vi "Configuration Files.vi"(8 "error in (no error)":errorcluster, 11 "Node Ptr":T3 format="%.0x") -> (0 "error out":errorcluster)   [LabVIEW 2020, in "Ballard ARINC 429 System Explorer.lvlib" / "Implementation.lvlib"]
uses:
  Implementation.lvlib
  <vilib>/NI VeriStand/Custom Device API/Custom Device Item Ref.ctl
  Types/Path Control.ctl
  Types/Browse Button.ctl
  Types/Configuration Files Page Data.ctl
  <vilib>/NI VeriStand/Custom Device API/Custom Device API.lvlib
  <vilib>/NI VeriStand/Custom Device Tools/Custom Device Utility Library/Custom Device Utility Library.lvlib
  Scripting/Ballard/Ballard ARINC 429 Scripting.lvlib
panel:
  in  "Refresh":bool
  in  "Parameters":T1
  in  "Hardware":T1
  in  "SHDocVw.IWebBrowser":refnum<k7>(container)
  in  "General Header":cluster{"Section Name":string}={"Section Name"="Ballard ARINC 429 - Configuration Files"}
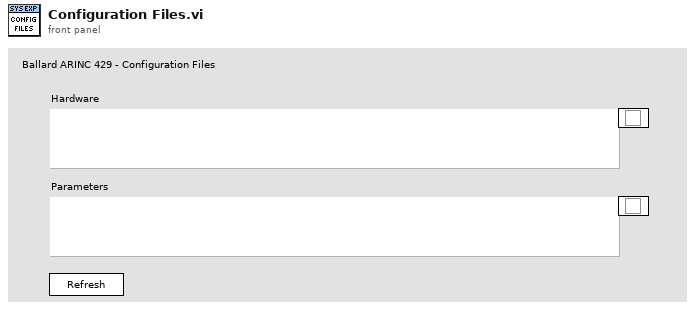
[diagram p1: front panel]
types:
  T1 = typedef "Ballard ARINC 429 System Explorer.lvlib/Implementation.lvlib/Path Control.ctl" = cluster{"file path":path, "Browse":T2}
  T2 = typedef "Ballard ARINC 429 System Explorer.lvlib/Implementation.lvlib/Browse Button.ctl" = bool
  T3 = typedef "Custom Device API.lvlib/Custom Device Item Ref.ctl" = u64
  T4 = typedef "Ballard ARINC 429 System Explorer.lvlib/Implementation.lvlib/Configuration Files Page Data.ctl" = cluster{"Hardware":T1, "Parameters":T1, "most recent parameters path":path, "most recent hardware path":path, "custom device ref":T3, "MD5 error":bool}
  T5 = typedef "Custom Device API.lvlib/Custom Device Commands.ctl" = enum16{"Default", "Item renamed", "Shutdown", "Dynamic button pressed"}
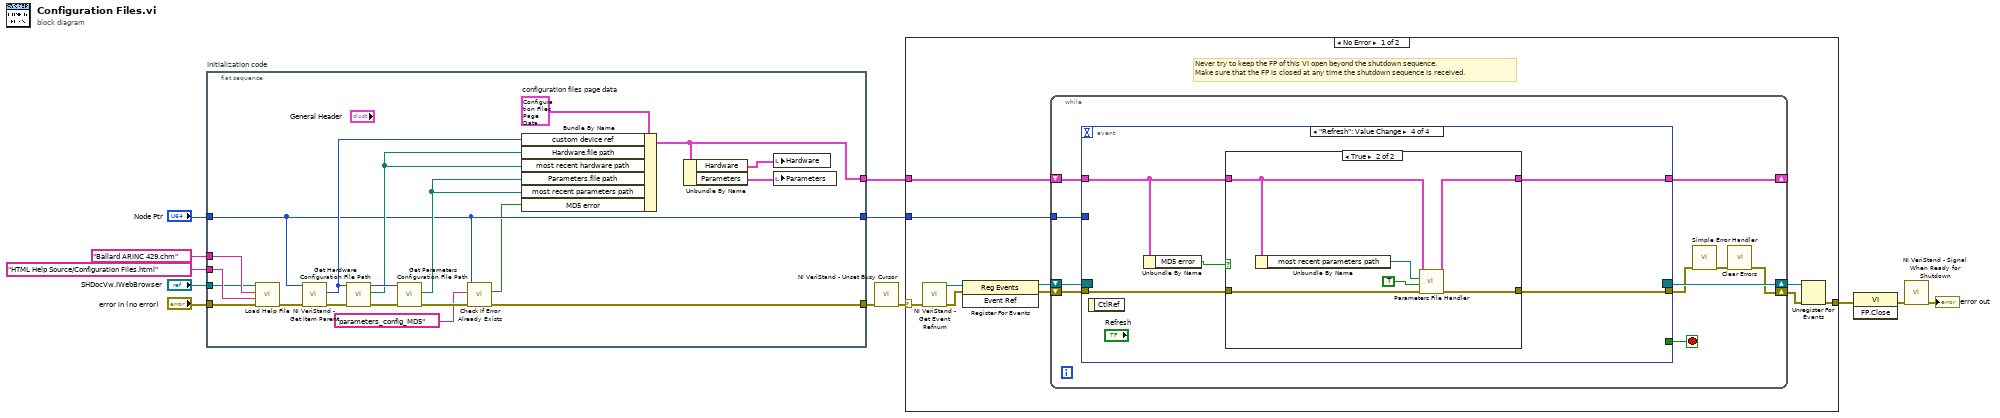
[diagram p0: block diagram]
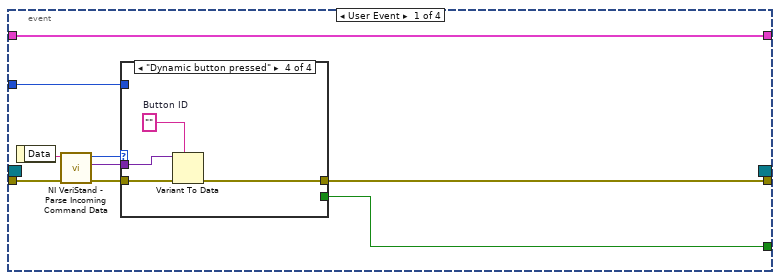
[diagram p2: hidden frame]
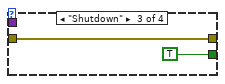
[diagram p5: hidden frame]
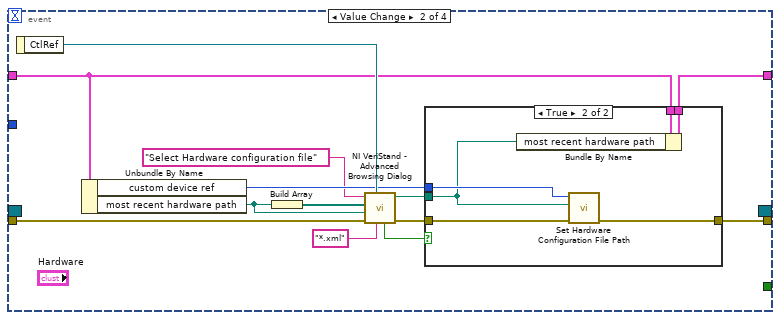
[diagram p6: hidden frame]
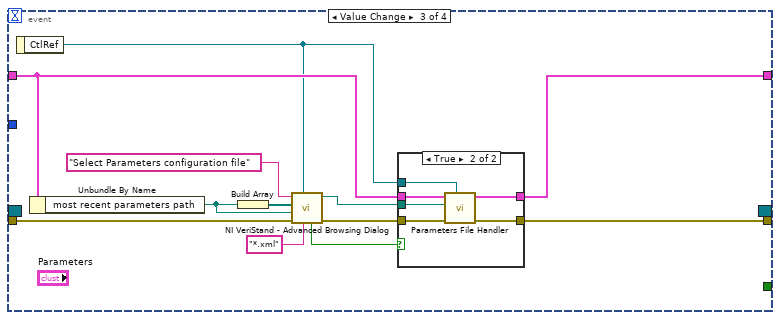
[diagram p8: hidden frame]
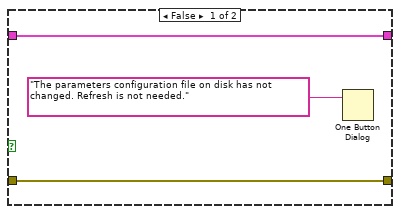
[diagram p10: hidden frame]
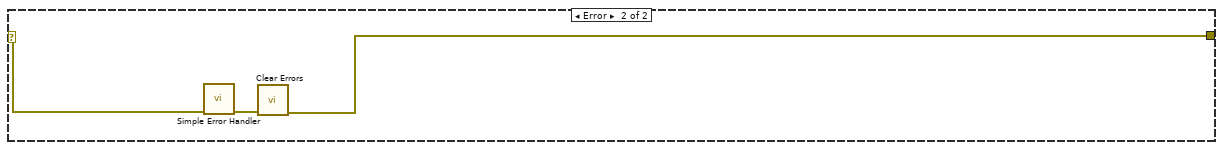
[diagram p11: hidden frame]
diagram:
  n1 = flat-sequence "Initialization code" {
    tunnel: "error in (no error)" -> [w32]
    tunnel: "Node Ptr" -> [w15]
    tunnel: [w16] -> w8
    tunnel: [w15] -> w5
    tunnel: "SHDocVw.IWebBrowser" -> [w20]
    tunnel: "HTML Help Source/Configuration Files.html" ("CD_CHM_Section") -> [w31]
    tunnel: "Ballard ARINC 429.chm" ("CD_CHM_FileName") -> [w30]
    tunnel: [w18] -> w1
    frame #0 {
      w29 = T4 {"Hardware"={"file path"=path "", "Browse"=FALSE}, "Parameters"={"file path"=path "", "Browse"=FALSE}, "most recent parameters path"=path "", "most recent hardware path"=path "", "custom device ref"=0, "MD5 error"=FALSE}  # configuration files page data
      n2 = call "Load Help File.vi"("error in (no error)"=w32, "HTML File to Load"=w31, "Main CHM File"=w30, "Browser"=w20) -> ("error out"=w23:errorcluster)  [unwired: 7 in]
      n3 = call <vilib>:"NI VeriStand - Get Item Parent.vi"("error in (no error)"=w23, "Item Ref in"=w15) -> ("error out"=w22:errorcluster, "Parent Ref"=w21:T3)  [unwired: 6 in, 2 out]
      n4 = call "Get Hardware Configuration File Path.vi"("error in"=w22, "custom device ref"=w21) -> ("error out"=w25:errorcluster, "path"=w24:path, "custom device ref out"=w26:T3)  [unwired: 6 in, 1 out]
      n5 = call "Get Parameters Configuration File Path.vi"("error in"=w25, "custom device ref"=w26) -> ("error out"=w17:errorcluster, "path"=w19:path)  [unwired: 6 in, 2 out]
      n6 = call "Check If Error Already Exists.vi"("error in"=w17, "error key"="parameters_config_MD5", "Configuration files Ref"=w15) -> ("error out"=w16:errorcluster, "error exists?"=w13:bool)  [unwired: 6 in, 1 out]
      n7 = Bundle By Name(cluster=w29, "custom device ref"=w21, "Hardware.file path"=w24, "most recent hardware path"=w24, "Parameters.file path"=w19, "most recent parameters path"=w19, "MD5 error"=w13) -> (w18:T4)
      n8 = Unbundle By Name(w18) -> ("Hardware"=w28:T1, "Parameters"=w27:T1)
      n9 = local write "Hardware"(w28) -> ()
      n10 = local write "Parameters"(w27) -> ()
    }
  }
  n11 = call <vilib>:"NI VeriStand - Unset Busy Cursor.vi"("error in (no error)"=w8) -> ("error out"=w7:errorcluster)  [unwired: 10 out]
  n12 = case shown="No Error" w7 {
    selector: w7 -> [w34 w127]
    tunnel: [w39 w125] -> w12
    tunnel: w5 -> [w35 _]
    tunnel: w1 -> [w33 _]
    frame No Error {
      # "Never try to keep the FP of this VI open beyond the shutdown sequence.\nMake sure that the FP is closed at any time the shutdown sequence is received."
      n13 = call <vilib>:"NI VeriStand - Get Event Refnum.vi"("error in (no error)"=w34) -> ("error out"=w42:errorcluster, "Event Ref"=w38:refnum<user-event>)  [unwired: 9 out]
      n14 = register-events(error in=w42, w38) -> (reference out=w36:refnum<event-registration>, error out=w37:errorcluster)  [unwired: 1 in]
      n15 = while {
        tunnel: w35 -> [w48]
        shift-right: [w45] -> w40
        shift-left: w37 -> [w51]
        shift-right: [w52] -> w41
        shift-left: w36 -> [w50]
        shift-right: [w43] -> _
        shift-left: w33 -> [w44]
        stop <- w49 stop-if-true
        n16 = event shown="[3] \"Refresh\": Value Change" {
          selector: w50 -> [_ _ _ _]
          dyn-events: [_ _ _ _] -> w52
          timeout: _ -> [_ _ _ _]
          tunnel: w51 -> [w61 w82 w102 w113]
          tunnel: [w57 _ _ _] -> w49
          tunnel: [w56 w76 w92 w114] -> w47
          tunnel: w48 -> [w55 _ _ _]
          tunnel: w44 -> [w53 w75 w96 w111]
          tunnel: [w53 w73 w95 w112] -> w43
          event User Event {
            n17 = event-data() -> ("Data"=w60:string)  [unwired: 1 out]
            n18 = call <vilib>:"NI VeriStand - Parse Incoming Command Data.vi"("error in (no error)"=w61, "Incoming data"=w60) -> ("error out"=w59:errorcluster, "Outgoing data"=w54:variant, "Action"=w58:T5)  [unwired: 7 out]
            n19 = case shown="\"Dynamic button pressed\"" w58 {
              tunnel: w59 -> [w62 w63 w64 w69]
              tunnel: [_ _ TRUE _] -> w57
              tunnel: [w62 w63 w64 w66] -> w56
              tunnel: w55 -> [_ _ _ _]
              tunnel: w54 -> [_ _ _ w68]
              frame "Default", Default {
              }
              frame "Item renamed" {
              }
              frame "Shutdown" {
              }
              frame "Dynamic button pressed" {
                w67 = ""  # Button ID
                n20 = Variant To Data(error in=w69, type=w67, Variant=w68) -> (error out=w66:errorcluster)  [unwired: 1 out]
              }
            }
          }
          event Value Change {
            n21 = event-data() -> ("CtlRef"=w80:refnum<vi>)  [unwired: 1 out]
            n22 = Unbundle By Name(w75) -> ("custom device ref"=w71:T3, "most recent hardware path"=w78:path)
            n23 = Build Array(w78) -> (w79:path[])
            n24 = call <vilib>:"NI VeriStand - Advanced Browsing Dialog.vi"("File Pattern"="*.xml", "CtlRef"=w80, "error in (no error)"=w82, "Most recent path"=w78, "Paths"=w79, "Dialog Title"="Select Hardware configuration file") -> ("error out"=w77:errorcluster, "Selected file"=w74:path, "Valid?"=w72:bool)  [unwired: 2 in, 1 out]
            n25 = case shown="True" w72 {
              tunnel: w77 -> [w84 w90]
              tunnel: w71 -> [_ w89]
              tunnel: [w84 w88] -> w76
              tunnel: w75 -> [w83 w87]
              tunnel: w74 -> [_ w86]
              tunnel: [w83 w85] -> w73
              frame False {
              }
              frame True {
                n26 = Bundle By Name(cluster=w87, "most recent hardware path"=w86) -> (w85:T4)
                n27 = call "Set Hardware Configuration File Path.vi"("error in"=w90, "path"=w86, "custom device ref"=w89) -> ("error out"=w88:errorcluster)  [unwired: 7 in, 1 out]
              }
            }
          }
          event Value Change {
            n28 = event-data() -> ("CtlRef"=w94:refnum<vi>)  [unwired: 1 out]
            n29 = Unbundle By Name(w96) -> ("most recent parameters path"=w98:path)
            n30 = Build Array(w98) -> (w100:path[])
            n31 = call <vilib>:"NI VeriStand - Advanced Browsing Dialog.vi"("File Pattern"="*.xml", "CtlRef"=w94, "error in (no error)"=w102, "Most recent path"=w98, "Paths"=w100, "Dialog Title"="Select Parameters configuration file") -> ("error out"=w97:errorcluster, "Selected file"=w93:path, "Valid?"=w91:bool)  [unwired: 2 in, 1 out]
            n32 = case shown="True" w91 {
              tunnel: w97 -> [w103 w110]
              tunnel: w96 -> [w104 w109]
              tunnel: [w104 w108] -> w95
              tunnel: w94 -> [_ w105]
              tunnel: w93 -> [_ w107]
              tunnel: [w103 w106] -> w92
              frame False {
              }
              frame True {
                n33 = call "Parameters File Handler.vi"("parameters path ctl ref"=w105, "error in"=w110, "selected parameters file"=w107, "configuration files page data"=w109) -> ("error out"=w106:errorcluster, "configuration files page data out"=w108:T4)  [unwired: 6 in]
              }
            }
          }
          event "Refresh": Value Change {
            n34 = event-data() -> ()  [unwired: 2 out]
            n35 = Unbundle By Name(w111) -> ("MD5 error"=w115:bool)
            n36 = case shown="True" w115 {
              tunnel: [w117 w124] -> w114
              tunnel: w113 -> [w117 w123]
              tunnel: w111 -> [w116 w122]
              tunnel: [w116 w120] -> w112
              frame False {
                n37 = One Button Dialog(message="The parameters configuration file on disk has not changed. Refresh is not needed.") -> ()  [unwired: 1 in, 1 out]
              }
              frame True {
                n38 = Unbundle By Name(w122) -> ("most recent parameters path"=w121:path)
                n39 = call "Parameters File Handler.vi"("error in"=w123, "refresh button"=TRUE, "selected parameters file"=w121, "configuration files page data"=w122) -> ("error out"=w124:errorcluster, "configuration files page data out"=w120:T4)  [unwired: 6 in]
              }
            }
          }
        }
        n40 = call <vilib>:"Simple Error Handler.vi"("error in (no error)"=w47) -> ("error out"=w46:errorcluster)  [unwired: 1 in, 7 out]
        n41 = call <vilib>:"Clear Errors.vi"("error in (no error)"=w46) -> ("error out"=w45:errorcluster)  [unwired: 1 in, 5 out]
      }
      n42 = Unregister For Events(event registration refnum=w41, error in=w40) -> (error out=w39:errorcluster)
    }
    frame Error {
      n43 = call <vilib>:"Simple Error Handler.vi"("error in (no error)"=w127) -> ("error out"=w126:errorcluster)  [unwired: 1 in, 7 out]
      n44 = call <vilib>:"Clear Errors.vi"("error in (no error)"=w126) -> ("error out"=w125:errorcluster)  [unwired: 1 in, 5 out]
    }
  }
  n45 = invoke class="VI" method="FP.Close"(error in=w12) -> (error out=w11:errorcluster)  [unwired: 2 in, 2 out]
  n46 = call <vilib>:"NI VeriStand - Signal When Ready for Shutdown.vi"("error in (no error)"=w11) -> ("error out"=→"error out":errorcluster)  [unwired: 10 out]
